vi "Disconnect.vi"(8 "error in (no error)":errorcluster, 11 "NRT8000 in":refnum<class "NRT8000.lvclass">) -> (0 "error out":errorcluster, 3 "NRT8000 out":refnum<class "NRT8000.lvclass">)   [LabVIEW 2018, in "NRT8000.lvlib" / "NRT8000.lvclass"]
uses:
  NRT8000.lvclass
  PPLs/Optical Spectrum Analyzer/Parent/OSA.lvlibp/Optical Spectrum Analyzer.lvclass
  C:/Projects/LabVIEW/PPLs/Optical Spectrum Analyzer/Parent/OSA.lvlibp/Optical Spectrum Analyzer.lvclass
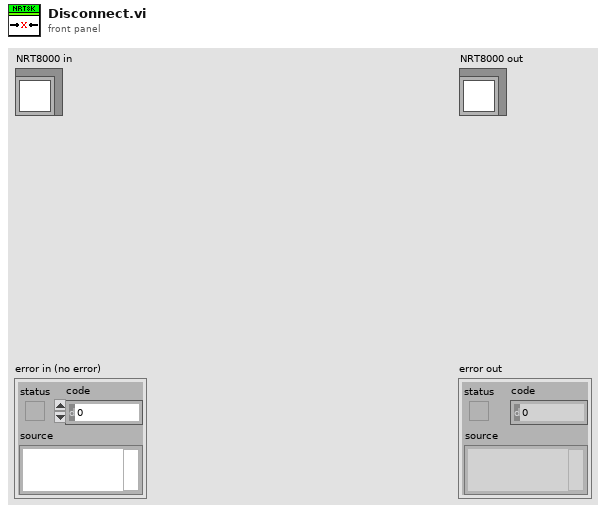
[diagram p1: front panel]
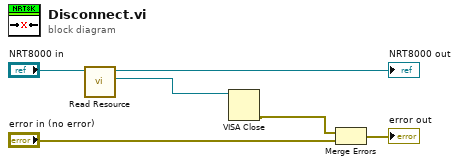
[diagram p0: block diagram]
diagram:
  n1 = call "Read Resource.vi"("Optical Spectrum Analyzer in"="NRT8000 in") -> ("Resource"=w2:refnum<visa-resource-name>, "Optical Spectrum Analyzer out"=→"NRT8000 out":refnum<class "NRT8000.lvclass">)  [unwired: 8 in, 1 out]
  n2 = VISA Close(VISA resource name=w2) -> (error out=w1:errorcluster)  [unwired: 1 in]
  n3 = Merge Errors(w1, "error in (no error)") -> (→"error out":errorcluster)
